vi "setSheetName.vi"(6 "Sheet Name":string, 8 "error in (no error)":errorcluster, 10 "SheetRef":refnum<k24>, 11 "MS-Excel in":refnum<class "MS-Excel.lvclass">) -> (0 "error out":errorcluster, 3 "MS-Excel out":refnum<class "MS-Excel.lvclass">)   [LabVIEW 2017, in "LabVIEW NPOI.lvlib" / "MS-Excel.lvclass"]
uses:
  MS-Excel.lvclass
  C:/Users/Neo/Desktop/Dev_Tools_BR/LabVIEW_NPOI/lib/NPOI 2.1.1/NPOI.dll
  lib/NPOI 2.1.1/NPOI.dll
  MS-Excel.lvclass/MS-Excel.ctl
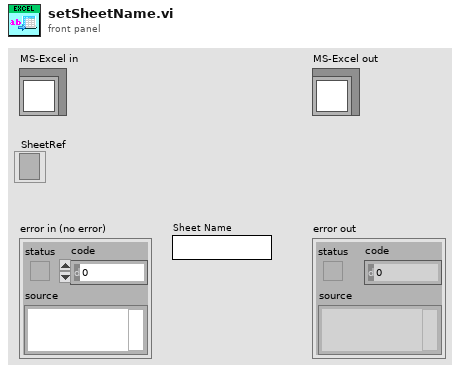
[diagram p1: front panel]
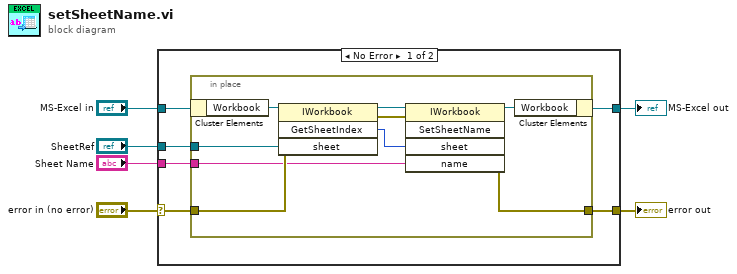
[diagram p0: block diagram]
diagram:
  n1 = case shown="No Error" "error in (no error)" {
    selector: "error in (no error)" -> [w10 w22]
    tunnel: [w9 w22] -> w6
    tunnel: [w12 w23] -> w4
    tunnel: "MS-Excel in" -> [w11 w23]
    tunnel: "Sheet Name" -> [w8 _]
    tunnel: "SheetRef" -> [w7 _]
    frame No Error {
      n2 = in-place {
        in-place-border: w10 -> [w19]
        in-place-border: [w13] -> w9
        in-place-border: w8 -> [w15]
        in-place-border: w7 -> [w18]
        n3 = in-place-cluster #1(w11) -> ("Workbook"=w21:refnum<k24>)
        n4 = invoke class="IWorkbook" method="GetSheetIndex"(reference=w21, error in=w19, "sheet"=w18) -> (reference out=w20:refnum<k24>, error out=w14:errorcluster, "GetSheetIndex"=w16:i32)  [unwired: 1 in, 1 out]
        n5 = invoke class="IWorkbook" method="SetSheetName"(reference=w20, error in=w14, "sheet"=w16, "name"=w15) -> (reference out=w17:refnum<k24>, error out=w13:errorcluster)  [unwired: 1 in, 3 out]
        n6 = in-place-cluster #1("Workbook"=w17) -> (w12:refnum<class "MS-Excel.lvclass">)
      }
    }
    frame Error {
    }
  }
  "error out" <- w6
  "MS-Excel out" <- w4
